vi "Helmholtz2D_Solve Lin Sys.vi"(5 "RHS":dbl[](array[numeric]), 6 "Boundary Condition":cluster{"type":T2, "Value":dbl[]}[](array[cluster]) {"type" items=["Dirichlet", "Neumann"]}, 7 "Domain":T3={"x"={"start x"=0.0, "end x"=1.0, "# of x-points"=11}, "y"={"start y"=0.0, "end y"=1.0, "# of y-points"=11}}, 8 "D":T1, 9 "C":T1, 10 "D'":T1, 11 "C'":T1) -> (3 "U(x, y)":dbl[][](array[numeric]))   [LabVIEW 2017, in "NI_PDE.lvlib"]
uses:
  <vilib>/gmath/NI_PDE.lvlib
  <vilib>/Analysis/Matrix/Datatypes/RealMatrix.ctl
  <vilib>/gmath/pde.llb/Common/PDE_BC Type.ctl
  <vilib>/Analysis/baseanly.llb/Real A x B.vi
  <vilib>/Analysis/baseanly.llb/A x Vector.vi
  <vilib>/Analysis/7linalg.llb/Solve Linear Equations (single right hand).vi
  <vilib>/Analysis/baseanly.llb/Solve Linear Equations By Cholesky.vi
  <vilib>/Analysis/baseanly.llb/Real Matrix to Compact Array.vi
  <vilib>/Analysis/baseanly.llb/Real Compact Tri-Matrix Linear Eqs.vi
  <vilib>/Analysis/baseanly.llb/Real Inverse Matrix.vi
  <vilib>/Analysis/Matrix/Numeric/Subtract/Subtract - RM,RM.vi
  <vilib>/Analysis/7linalg.llb/Solve Linear Eqs (General).vi
  <vilib>/Analysis/7linalg.llb/Solve Linear Eqs (Gen, single right hand).vi
  <vilib>/Analysis/NI_AALBase.lvlib
  <vilib>/Analysis/Matrix/NI_Matrix.lvlib
  <vilib>/Analysis/NI_AALPro.lvlib
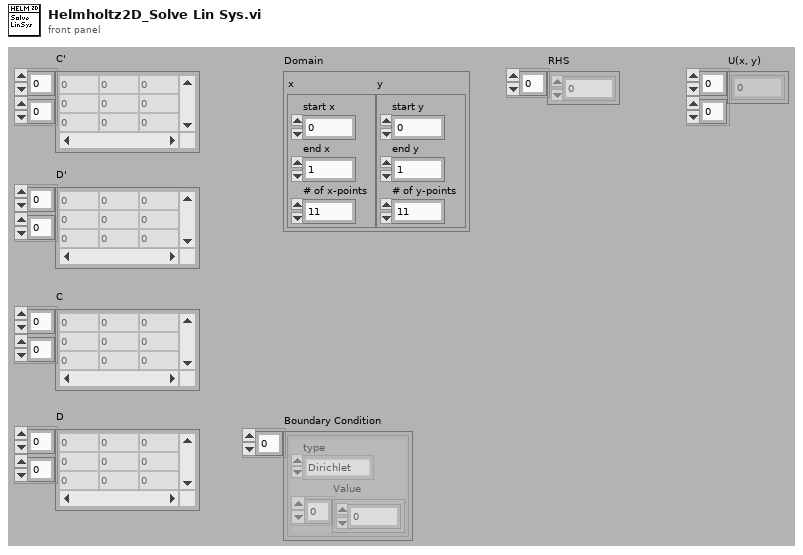
[diagram p1: front panel]
types:
  T1 = typedef "NI_Matrix.lvlib/RealMatrix.ctl" = dbl[][]
  T2 = typedef "NI_PDE.lvlib/PDE_BC Type.ctl" = i32
  T3 = cluster{"x":cluster{"start x":dbl, "end x":dbl, "# of x-points":i32}, "y":cluster{"start y":dbl, "end y":dbl, "# of y-points":i32}}
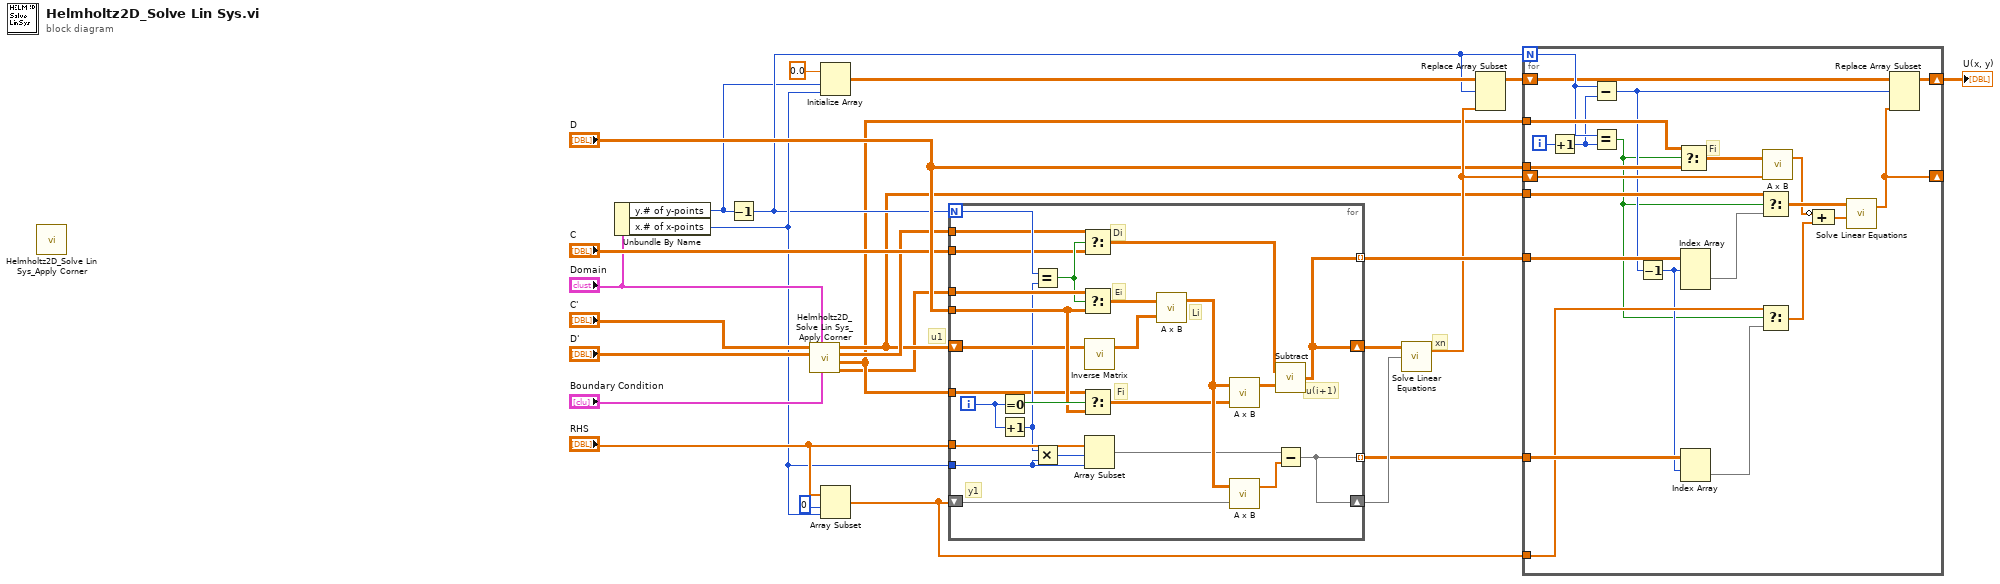
[diagram p0: block diagram]
diagram:
  # "xn"
  # "u1"
  n1 = call <vilib>:"Helmholtz2D_Solve Lin Sys_Apply Corner.vi"() -> ()  [unwired: 4 in, 8 out]
  n2 = Unbundle By Name("Domain") -> ("y.# of y-points"=w5:i32, "x.# of x-points"=w7:i32)
  n3 = Decrement(x=w5) -> (x-1=w6:i32)
  n4 = call <vilib>:"Helmholtz2D_Solve Lin Sys_Apply Corner.vi"("Boundary Condition"="Boundary Condition", "Domain"="Domain", "D"="D'", "C'"="C'") -> ("D' End Y"=w1:T1, "D' Start Y"=w2:T1, "C' End Y"=w4:T1, "C' Start Y"=w3:T1)  [unwired: 4 out]
  n5 = Initialize Array(0.0 ("element"), w5, w7) -> (w17:dbl[][])
  n6 = Array Subset(array="RHS", index=0, length=w7) -> (w16:dbl[])
  n7 = for {
    N: w6 -> [w49]
    shift-right: [w29] -> w24
    shift-left: w3 -> [w45]
    tunnel: "RHS" -> [w50]
    tunnel: "D" -> [w46]
    tunnel: w1 -> [w47]
    tunnel: "C" -> [w40]
    tunnel: w4 -> [w39]
    shift-right: [w31] -> w23
    shift-left: w16 -> [w36]
    tunnel: [w31] -> w22 mode=indexing
    tunnel: [w29] -> w21 mode=indexing
    tunnel: w7 -> [w28]
    tunnel: w2 -> [w27]
    i -> [w35]
    # "y1"
    # "u(i+1)"
    # "Di"
    # "Ei"
    # "Fi"
    # "Li"
    n8 = Equal To 0?(x=w35) -> (x = 0?=w48:bool)
    n9 = Increment(x=w35) -> (x+1=w34:i32)
    n10 = Equal?(x=w49, y=w34) -> (x = y?=w41:bool)
    n11 = Multiply(x=w34, y=w28) -> (x*y=w26:i32)
    n12 = Select(t=w39, s=w41, f=w40) -> (s? t:f=w38:T1)
    n13 = Select(t=w47, s=w41, f=w46) -> (s? t:f=w43:T1)
    n14 = Select(t=w27, s=w48, f=w46) -> (s? t:f=w30:T1)
    n15 = call-poly <vilib>:"Inverse Matrix.vi"("Input Matrix"=w45) -> ("Inverse Matrix"=w44:T1)  [unwired: 1 in, 1 out]
    n16 = Array Subset(array=w50, index=w26, length=w28) -> (w33:dbl[])
    n17 = call-poly <vilib>:"A x B.vi"("B"=w44, "A"=w43) -> ("A x B"=w37:T1)  [unwired: 1 out]
    n18 = call-poly <vilib>:"A x B.vi"("B"=w30, "A"=w37) -> ("A x B"=w42:T1)  [unwired: 1 out]
    n19 = call-poly <vilib>:"A x B.vi"("Vector"=w36, "A"=w37) -> ("A x Vector"=w32:dbl[])  [unwired: 1 out]
    n20 = call-poly <vilib>:"Subtract.vi"("Real Matrix B"=w42, "Real Matrix A"=w38) -> ("A - B"=w29:T1)
    n21 = Subtract(x=w33, y=w32) -> (x-y=w31:dbl[])
  }
  n22 = call-poly <vilib>:"Solve Linear Equations.vi"("Known Vector"=w23, "Input Matrix"=w24) -> ("Solution Vector"=w19:dbl[])  [unwired: 1 in, 1 out]
  n23 = Replace Array Subset(array=w17, new element=w19, index (row)=w6) -> (w20:dbl[][])  [unwired: 1 in]
  n24 = for {
    N: w6 -> [w67]
    tunnel: w22 -> [w68]
    tunnel: w21 -> [w63]
    shift-right: [w56] -> _
    shift-left: w19 -> [w73]
    tunnel: "D" -> [w71]
    tunnel: w2 -> [w69]
    tunnel: w16 -> [w64]
    tunnel: w3 -> [w59]
    shift-right: [w57] -> w15
    shift-left: w20 -> [w58]
    i -> [w72]
    # "Fi"
    n25 = Increment(x=w72) -> (x+1=w66:i32)
    n26 = Subtract(x=w67, y=w66) -> (x-y=w55:i32)
    n27 = Equal?(x=w67, y=w66) -> (x = y?=w54:bool)
    n28 = Decrement(x=w55) -> (x-1=w62:i32)
    n29 = Select(t=w69, s=w54, f=w71) -> (s? t:f=w70:T1)
    n30 = Index Array(array=w63, index (dim 0)=w62) -> (element=w60:dbl[][])  [unwired: 2 in]
    n31 = Index Array(array=w68, index (row)=w62) -> (element=w65:dbl[])  [unwired: 1 in]
    n32 = Select(t=w59, s=w54, f=w60) -> (s? t:f=w61:dbl[][])
    n33 = Select(t=w64, s=w54, f=w65) -> (s? t:f=w53:dbl[])
    n34 = call-poly <vilib>:"A x B.vi"("Vector"=w73, "A"=w70) -> ("A x Vector"=w51:dbl[])  [unwired: 1 out]
    n35 = Compound Arithmetic op=ADD(invert w51, w53) -> (w52:dbl[])
    n36 = call-poly <vilib>:"Solve Linear Equations.vi"("Known Vector"=w52, "Input Matrix"=w61) -> ("Solution Vector"=w56:dbl[])  [unwired: 1 in, 1 out]
    n37 = Replace Array Subset(array=w58, new element=w56, index (row)=w55) -> (w57:dbl[][])  [unwired: 1 in]
  }
  "U(x, y)" <- w15
